vi "Fined Pupil With Circular Edge.vi"(7 "error in":errorcluster) -> (27 "error out":errorcluster)   [LabVIEW 2015]
panel:
  out "Fitted Circle":T1 {"Average SNR (dB)" format="%.2f"; "Average Strength" format="%.2f"; "Roundness (Real-World)" format="%.2f"; "Radius (Real-World)" format="%.2f"; "Center (Real-World)"."Y" format="%.2f"; "Center (Real-World)"."X" format="%.2f"; "Radius (Pixels)" format="%.2f"; "Center (Pixels)"."Y" format="%.2f"; "Center (Pixels)"."X" format="%.2f"}
  out "Image Out":T2(plugin-control)
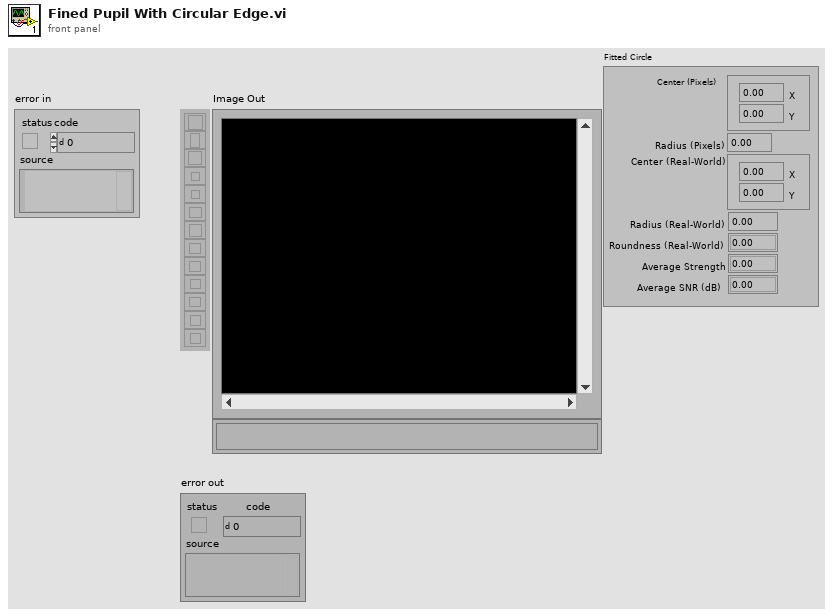
[diagram p1: front panel]
types:
  T1 = cluster{"Center (Pixels)":cluster{"X":sgl, "Y":sgl}, "Radius (Pixels)":dbl, "Center (Real-World)":cluster{"X":sgl, "Y":sgl}, "Radius (Real-World)":dbl, "Roundness (Real-World)":dbl, "Average Strength":dbl, "Average SNR (dB)":dbl}
  T2 = typedef "IMAQ Image.ctl" = refnum<image>
  T3 = typedef "Image Type" = u32
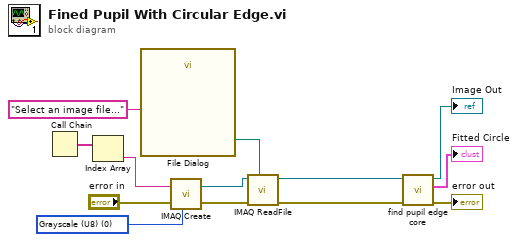
[diagram p0: block diagram]
diagram:
  w6 = T3 0 items=["Grayscale (U8)", "Grayscale (I16)", "Grayscale (SGL)", "Complex (CSG)", "RGB (U32)", "HSL (U32)", "RGB (U64)", "Grayscale (U16)"] ("Image Type")
  n1 = Call Chain() -> (call chain=w10:string[])
  n2 = Index Array(array=w10) -> (element=w9:string)  [unwired: 1 in]
  n3 = call "File Dialog"("prompt"="Select an image file...") -> ("selected path"=w7:path)  [unwired: 6 in, 8 out]
  n4 = call "IMAQ Create"("Image Name"=w9, "Image Type"=w6, "error in (no error)"="error in") -> ("New Image"=w13:T2, "error out"=w12:errorcluster)  [unwired: 1 in, 1 out]
  n5 = call "IMAQ ReadFile"("File Path"=w7, "error in (no error)"=w12, "Image"=w13) -> ("error out"=w4:errorcluster, "Image Out"=w5:T2)  [unwired: 2 in, 5 out]
  n6 = call "find pupil edge core.vi"("error in (no error)"=w4, "Refnum in"=w5) -> ("error out"=→"error out":errorcluster, "Fitted Circle"=→"Fitted Circle":T1, "Refnum out"=→"Image Out":T2)  [unwired: 7 in]
